vi "FFT UI.vi"() -> ()   [LabVIEW 2014]
doc: "This VI provides a UI for the \"LabVIEW FPGA FFT.vi\" example."
uses:
  <vilib>/FPGAPlugInAG/sbRIO-9636/niLvFpga_Open_sbRIO-9636.vi
  <vilib>/rvi/interface/common/dynamic/niFpgaDynamicAddResources.vi
  <vilib>/rvi/Analysis/host/Private/Sample Rate To Loop Time (ticks).vi
  <vilib>/Utility/error.llb/Error Cluster From Error Code.vi
  <vilib>/rvi/errors/niLvFpgaAdjustHostInterfaceError.vi
  <vilib>/FPGAPlugInAG/Dynamic/niLvFpga_Close_Dynamic.vi
  <vilib>/rvi/interface/nirviOpenFPGA/nirviOpenFPGA.xnode
  FPGA Bitfiles/FFT_FPGATarget_LabVIEWFPGAFFT_5PZwCVPO07s.lvbitx
  LabVIEW FPGA FFT.vi
  <vilib>/rvi/interface/nirviReadWriteControl/nirviReadWriteControl.xnode
  <vilib>/rvi/interface/nirviMethod/nirviMethod.xnode
  <vilib>/rvi/interface/nirviCloseFPGA/nirviCloseFPGA.xnode
  <vilib>/rvi/Analysis/host/Public/NI_FpgaMspHost.lvlib
  <vilib>/FPGAPlugInAG/Dynamic/niLvFpga_ReadFifo_Dynamic.vi
  <vilib>/rvi/errors/niLvFpgaMergeErrorWithErrorCode.vi
  NiFpgaLv.dll
  <vilib>/rvi/interface/Simulation/niFpgaSimulationCallBeginRW.vi
panel:
  out "Signal":waveform(dbl)(graph)={"t0"=timestamp(0 s since 1904-01-01), "dt"=2e-05, "Y"=[]}
  out "FFT Spectrum":waveform(dbl)(graph)={"t0"=timestamp(0 s since 1904-01-01), "dt"=195.3125, "Y"=[]}
  in  "Stop":bool
  in  "Frequency (Hz)":dbl=4000.0 min=0.0 format="%#_7p"
  in  "Sample rate (S/s)":dbl=50000.0 min=1.0 format="%#_7p"
  out "Invalid Sample Rate":bool
  # "Overview: Demonstrates the use of the LabVIEW FPGA FFT function for custom in-hardware signal processing\nRequirements: LabVIEW FPGA Module, NI-RIO\nInstructions: Run the VI"
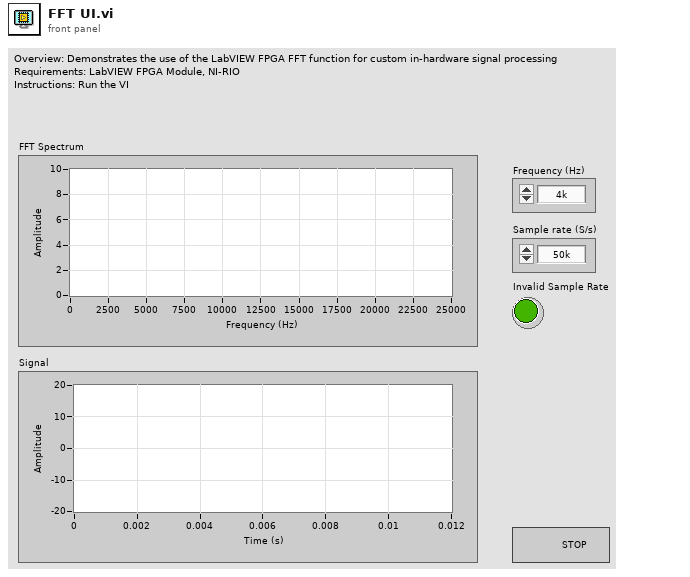
[diagram p1: front panel]
types:
  T1 = typedef "niFpgaViExecutionMode.ctl" = enum16{"FPGA Target", "Simulation (Simulated I/O)", "Simulation (Real I/O)", "Third-Party Simulation"}
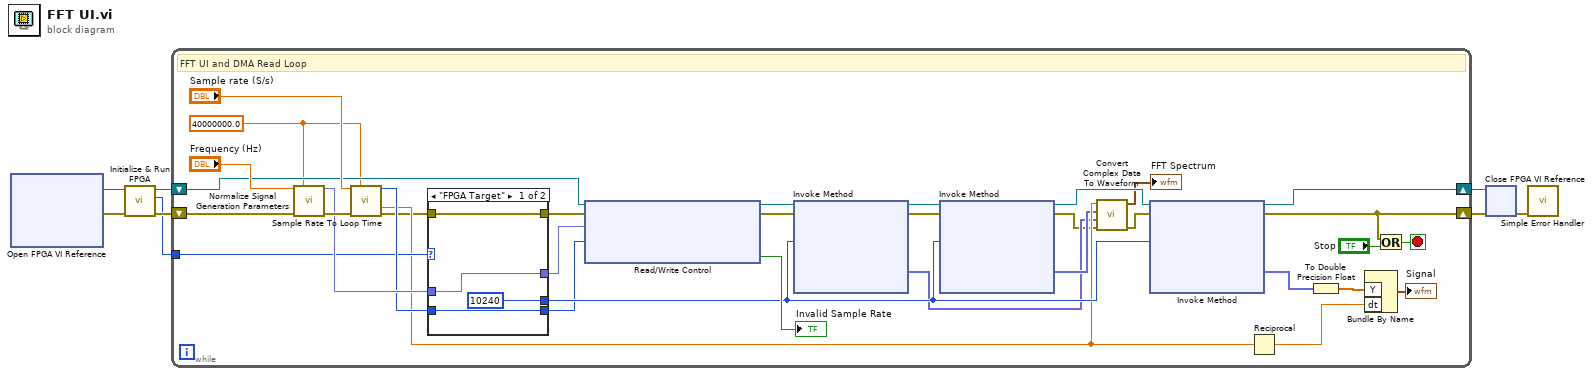
[diagram p0: block diagram]
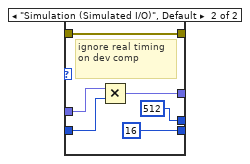
[diagram p2: hidden frame]
diagram:
  n1 = xnode "Open FPGA VI Reference"() -> ("FPGA VI Reference Out"=w3:refnum<k20>, "error out"=w2:errorcluster)  [unwired: 2 in]
  n2 = call "Initialize & Run FPGA.vi"("error in (no error)"=w2, "Refnum in"=w3) -> ("error out"=w5:errorcluster, "FPGA VI Execution Mode"=w4:T1, "Refnum out"=w6:refnum<k20>)  [unwired: 7 in]
  n3 = while {
    shift-right: [w39] -> w8
    shift-left: w6 -> [w21]
    shift-right: [w23] -> w7
    shift-left: w5 -> [w22]
    tunnel: w4 -> [w18]
    stop <- w33 stop-if-true
    w20 = 40000000.0 ("FPGA clock rate (Hz)")
    # "FFT UI and DMA Read Loop"
    n4 = call <vilib>:"Normalize Signal Generation Parameters.vi"("frequency (Hz)"="Frequency (Hz)", "FPGA clock rate (Hz)"=w20, "error in (no error)"=w22) -> ("frequency (periods/tick)"=w37:fxp<+,32,0>, "error out"=w38:errorcluster)  [unwired: 11 in]
    n5 = call-poly <vilib>:"Sample Rate To Loop Time.vi"("sample rate (S/s)"="Sample rate (S/s)", "FPGA clock rate (Hz)"=w20, "error in (no error)"=w38) -> ("count (ticks/S)"=w32:u32, "actual sample rate (S/s)"=w17:dbl, "error out"=w12:errorcluster)  [unwired: 10 in]
    n6 = case shown="\"FPGA Target\"" w18 {
      tunnel: [u32 10240 ("Number of Elements") u32 512 ("Number of Elements")] -> w26
      tunnel: w37 -> [w45 w51]
      tunnel: [w45 w50] -> w28
      tunnel: w32 -> [w44 w49]
      tunnel: [w44 u32 16 ("count (ticks/S)")] -> w19
      tunnel: w12 -> [w43 w47]
      tunnel: [w43 w47] -> w11
      frame "FPGA Target" {
      }
      frame "Simulation (Simulated I/O)", Default {
        # "ignore real timing on dev comp"
        n7 = Multiply(x=w51, y=w49) -> (x*y=w50:fxp<+,32,0>)
      }
    }
    n8 = xnode "Read/Write Control"("FPGA VI Reference In"=w21, "error in"=w11, "Frequency (periods/tick)"=w28, "Requested Sample Period (ticks)"=w19) -> ("FPGA VI Reference Out"=w31:refnum<k20>, "error out"=w24:errorcluster, "Invalid Period"=→"Invalid Sample Rate":bool)
    n9 = xnode "Invoke Method"("FPGA VI Reference In"=w31, "error in"=w24, "Number of Elements"=w26) -> ("FPGA VI Reference Out"=w41:refnum<k20>, "error out"=w25:errorcluster, "Data"=w15:fxp<+/-,25,14>[])  [unwired: 1 in, 1 out]
    n10 = xnode "Invoke Method"("FPGA VI Reference In"=w41, "error in"=w25, "Number of Elements"=w26) -> ("FPGA VI Reference Out"=w40:refnum<k20>, "error out"=w14:errorcluster, "Data"=w16:fxp<+/-,25,14>[])  [unwired: 1 in, 1 out]
    n11 = call "Convert Complex Data To Waveform.vi"("error in"=w14, "Real Data"=w15, "Imaginary Data"=w16, "Sample Rate (S/s)"=w17) -> ("error out"=w13:errorcluster, "Waveform"=→"FFT Spectrum":waveform(dbl))  [unwired: 6 in]
    n12 = xnode "Invoke Method"("FPGA VI Reference In"=w40, "error in"=w13, "Number of Elements"=w26) -> ("FPGA VI Reference Out"=w39:refnum<k20>, "error out"=w23:errorcluster, "Data"=w42:fxp<+/-,16,5>[])  [unwired: 1 in, 1 out]
    n13 = Reciprocal(x=w17) -> (1/x=w35:dbl)
    n14 = To Double Precision Float(number=w42) -> (double precision float=w36:dbl[])
    n15 = Bundle By Name("Y"=w36, "dt"=w35) -> (→"Signal":waveform(dbl))  [unwired: 1 in]
    n16 = Or(x=w23, y="Stop") -> (x .or. y?=w33:bool)
  }
  n17 = xnode "Close FPGA VI Reference"("FPGA VI Reference In"=w8, "error in"=w7) -> ("error out"=w1:errorcluster)
  n18 = call <vilib>:"Simple Error Handler.vi"("error in (no error)"=w1) -> ()  [unwired: 4 in, 5 out]
